vi "Enum Value.vi"(10 "Enumeration":T1) -> (2 "Value":i32)   [LabVIEW 2020, in "ConnectStatus.lvlib"]
uses:
  ConnectStatus.lvlib
  Enumeration.ctl
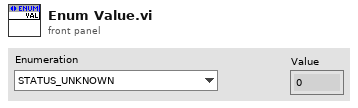
[diagram p1: front panel]
types:
  T1 = typedef "ConnectStatus.lvlib/Enumeration.ctl" = enum16{"STATUS_UNKNOWN", "STATUS_SUCCESS", "STATUS_ERROR", "STATUS_BAD_CONFIG", "STATUS_BAD_SYSTEM", "STATUS_BAD_CLUSTER"}
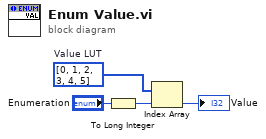
[diagram p0: block diagram]
diagram:
  w4 = i32[] [0, 1, 2, 3, 4, 5]  # Value LUT
  n1 = To Long Integer(number="Enumeration") -> (32bit integer=w1:i32)
  n2 = Index Array(array=w4, index=w1) -> (element=→"Value":i32)
